vi "Initialization VI.vi"(8 "error in (no error)":errorcluster, 10 "Custom XML":string, 11 "Device Item Ref in":T1 format="%.0x") -> (0 "error out":errorcluster, 3 "Device Item Ref out":T1 format="%.0x")   [LabVIEW 2015, in "DMM-SWITCH-ScanList System Explorer.lvlib"]
uses:
  DMM-SWITCH-ScanList System Explorer.lvlib
  <vilib>/NI Veristand/Custom Device API/Custom Device Item Ref.ctl
  <instrlib>/niDMM/nidmm.llb/niDMM Function.ctl
  <instrlib>/niDMM/nidmm.llb/niDMM Resolution in Digits.ctl
  <instrlib>/niSwitch/niSwitch.LLB/niSwitch Topologies.ctl
  <instrlib>/niSwitch/niSwitch.LLB/niSwitch Trigger Input.ctl
  <instrlib>/niSwitch/niSwitch.LLB/niSwitch Scan Advanced Output.ctl
  <instrlib>/niDMM/nidmm.llb/niDMM Measurement Complete.ctl
  <instrlib>/niDMM/nidmm.llb/niDMM Trigger.ctl
  <vilib>/NI Veristand/Custom Device API/Custom Device Channel.ctl
  <vilib>/NI Veristand/Custom Device API/Custom Device Channel Type.ctl
  Shared/Constants.vi
  <vilib>/NI Veristand/Custom Device API/Custom Device API.lvlib
  Shared/DMM-SWITCH-ScanList Shared.lvlib
  <vilib>/NI/Configuration Framework/serializable configuration/NISE_CEF_serializable configuration.lvclass
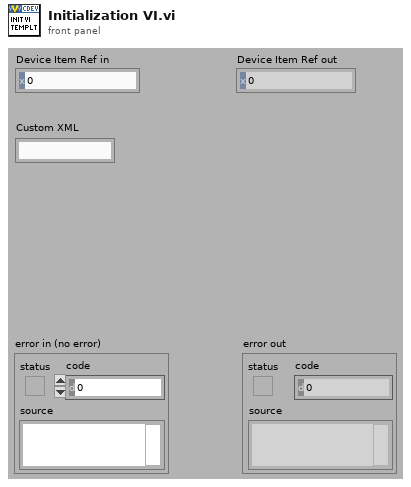
[diagram p1: front panel]
types:
  T1 = typedef "Custom Device API.lvlib/Custom Device Item Ref.ctl" = u64
  T2 = typedef "niDMM Trigger.ctl" = enum16{"Immediate", "External", "TTL 0", "TTL 1", "TTL 2", "TTL 3", "TTL 4", "TTL 5", "TTL 6", "Software", "TTL 7", "PXI Star", "LBR Trig 1", "Aux Trig 1"}
  T3 = typedef "niDMM Measurement Complete.ctl" = enum16{"None", "External", "TTL 0", "TTL 1", "TTL 2", "TTL 3", "TTL 4", "TTL 5", "TTL 6", "TTL 7", "LBR Trig 0"}
  T4 = typedef "niSwitch Scan Advanced Output.ctl" = enum16{"None", "External", "TTL0", "TTL1", "TTL2", "TTL3", "TTL4", "TTL5", "TTL6", "TTL7", "ECL0", "ECL1", "PXI Star", "Rear Connector", "Front Connector", "Rear Connector Module 1", "Rear Connector Module 2", "Rear Connector Module 3", "Rear Connector Module 4", "Rear Connector Module 5", "Rear Connector Module 6", "Rear Connector Module 7", "Rear Connector Module 8", "Rear Connector Module 9", "Rear Connector Module 10", "Rear Connector Module 11", "Rear Connector Module 12", "Front Connector Module 1", "Front Connector Module 2", "Front Connector Module 3", "Front Connector Module 4", "Front Connector Module 5", "Front Connector Module 6", "Front Connector Module 7", "Front Connector Module 8", "Front Connector Module 9", "Front Connector Module 10", "Front Connector Module 11", "Front Connector Module 12"}
  T5 = typedef "niSwitch Trigger Input.ctl" = enum16{"Immediate", "External", "TTL0", "TTL1", "TTL2", "TTL3", "TTL4", "TTL5", "TTL6", "TTL7", "ECL0", "ECL1", "PXI Star", "Software Trigger Function", "Rear Connector", "Front Connector", "Rear Connector of Module 1", "Rear Connector of Module 2", "Rear Connector of Module 3", "Rear Connector of Module 4", "Rear Connector of Module 5", "Rear Connector of Module 6", "Rear Connector of Module 7", "Rear Connector of Module 8", "Rear Connector of Module 9", "Rear Connector of Module 10", "Rear Connector of Module 11", "Rear Connector of Module 12", "Front Connector of Module 1", "Front Connector of Module 2", "Front Connector of Module 3", "Front Connector of Module 4", "Front Connector of Module 5", "Front Connector of Module 6", "Front Connector of Module 7", "Front Connector of Module 8", "Front Connector of Module 9", "Front Connector of Module 10", "Front Connector of Module 11", "Front Connector of Module 12"}
  T6 = typedef "niDMM Function.ctl" = enum16{"DC Volts", "AC Volts", "DC Current", "AC Current", "2-wire Resistance", "4-wire Resistance", "Diode", "Frequency", "Period", "AC Volts DC Coupled", "Capacitance", "Inductance", "Temperature"}
  T7 = typedef "niSwitch Topologies.ctl" = string
  T8 = typedef "niDMM Resolution in Digits.ctl" = dbl
  T9 = typedef "Custom Device API.lvlib/Custom Device Channel.ctl" = cluster{"Type":T10, "Units":string, "Default Value":dbl, "Faultable":bool, "Scalable":bool}
  T10 = typedef "Custom Device API.lvlib/Custom Device Channel Type.ctl" = enum16{"Input", "Output"}
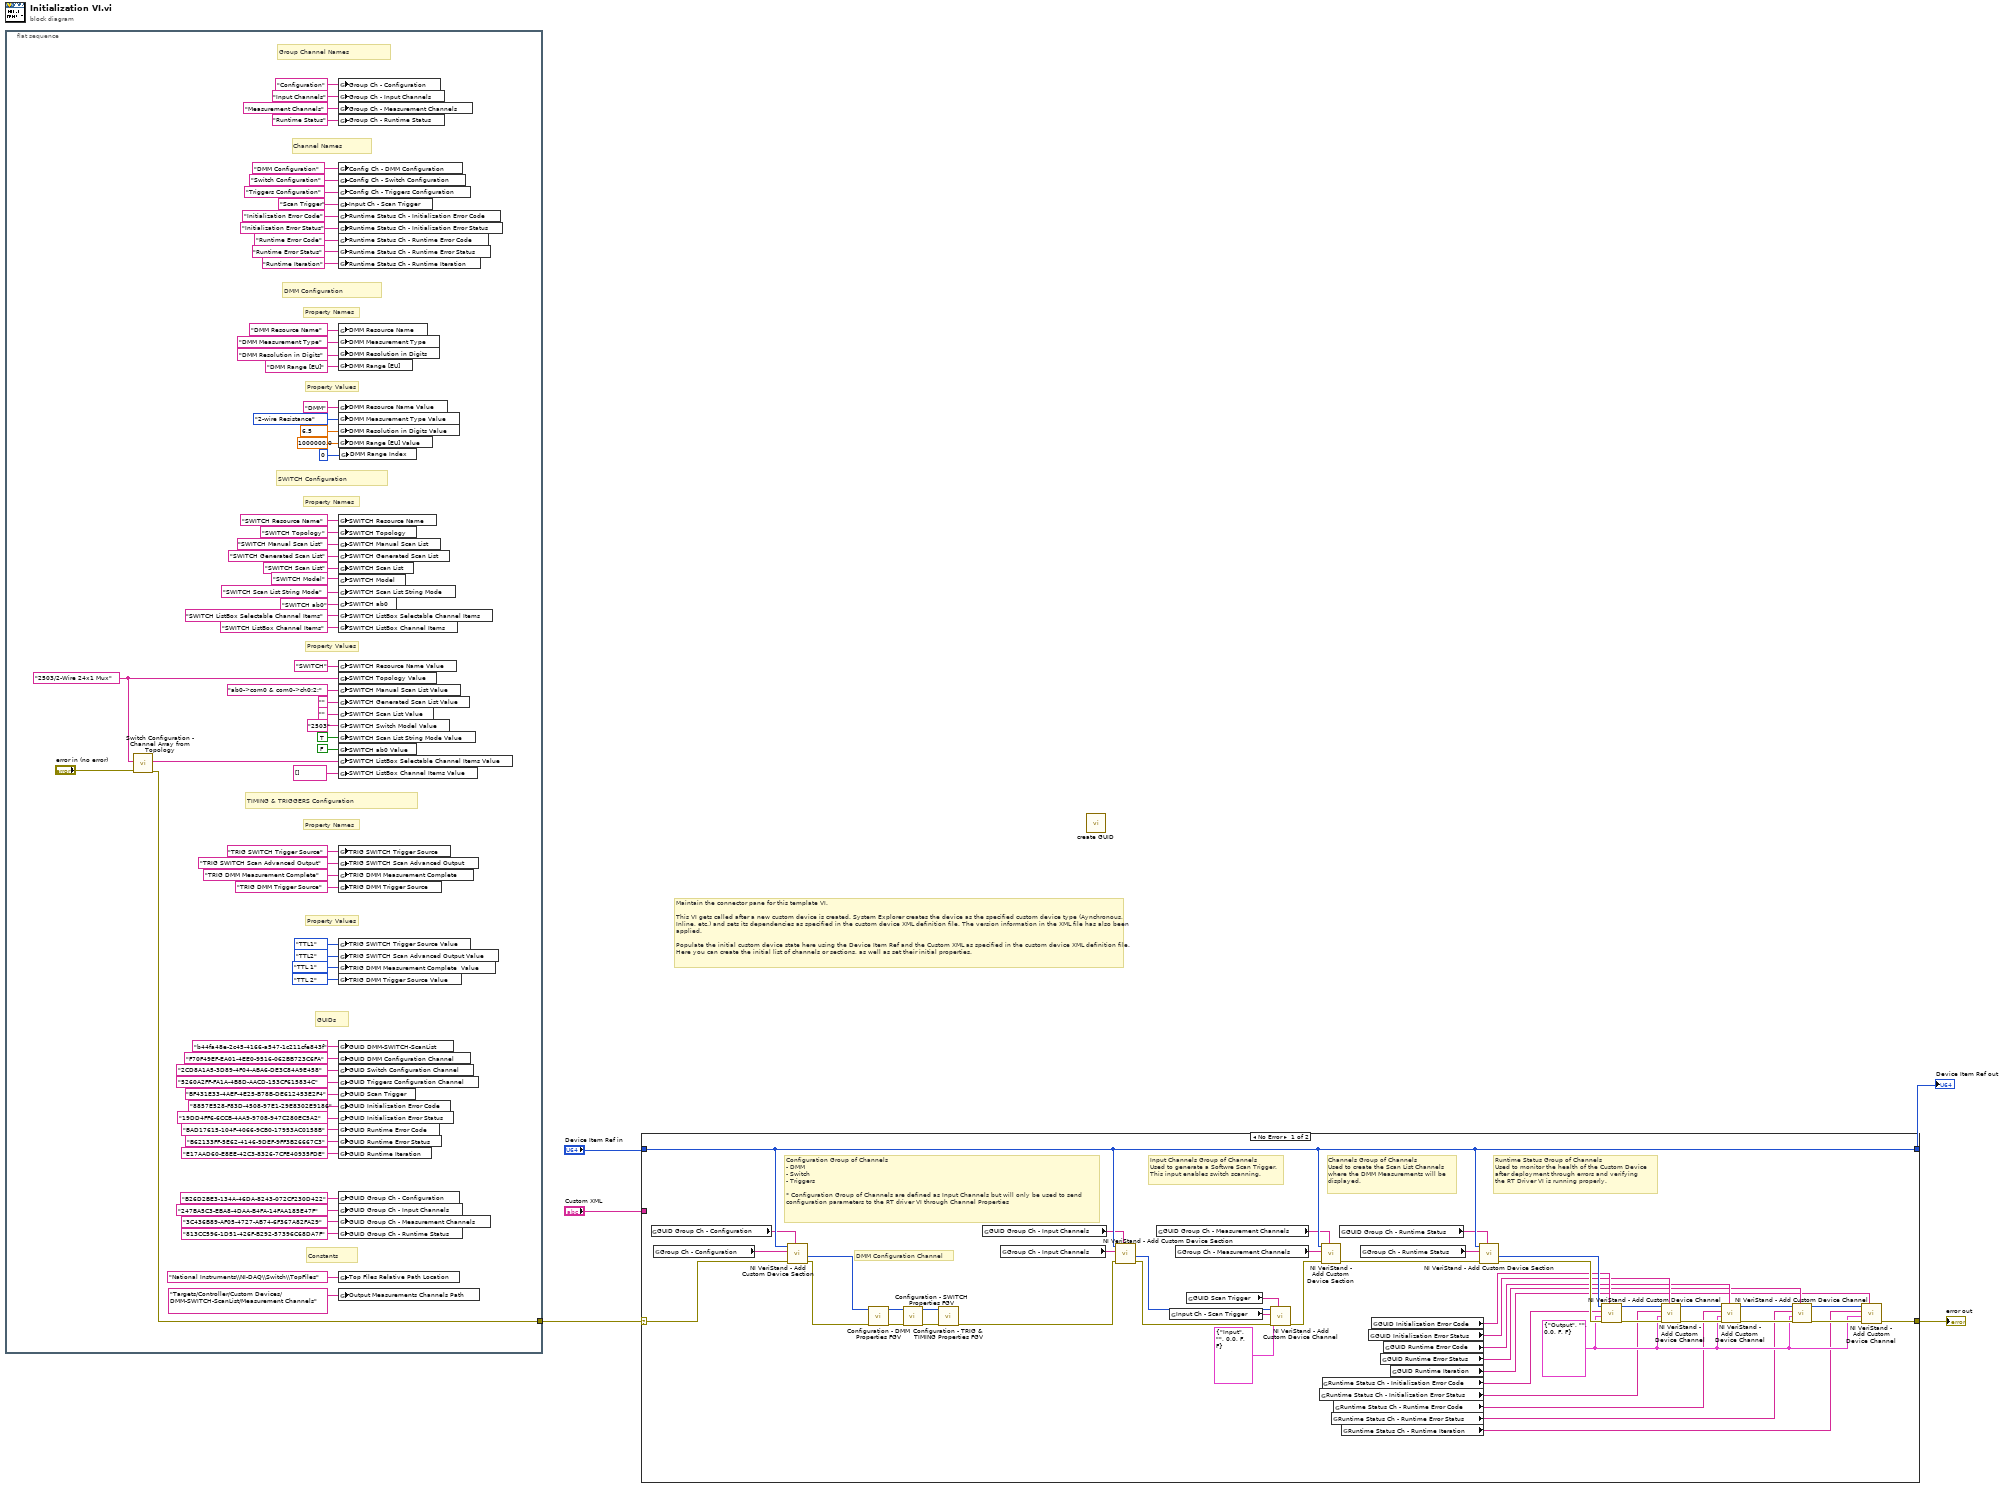
[diagram p0: block diagram]
diagram:
  # "Maintain the connector pane for this template VI.\n\nThis VI gets called after a new custom device is created. System Explorer creates the device as the specified custom device type (Aynchronous, Inline, etc.) and sets its dependencies as specified in the custom device XML definition file. The version information in the XML file has also been applied.\n\nPopulate the initial custom device state here using the Device Item Ref and the Custom XML as specified in the custom device XML definition file. Here you can create the initial list of channels or sections, as well as set their initial properties."
  n1 = flat-sequence {
    tunnel: [w54] -> w5
    frame #0 {
      w55 = T7 "2503/2-Wire 24x1 Mux" ("SWITCH Topology")
      w71 = T8 6.5 items=["3 1/2"=3.5, "4 1/2"=4.5, "5 1/2"=5.5, "6 1/2"=6.5, "7 1/2"=7.5] ("Resolution in Digits")
      # "Channel Names"
      # "Group Channel Names"
      # "Property Values"
      # "Property Names"
      # "Property Values"
      # "Property Names"
      # "Property Values"
      # "Property Names"
      # "Constants"
      # "DMM Configuration"
      # "GUIDs"
      # "TIMING & TRIGGERS Configuration"
      # "SWITCH Configuration"
      n2 = call "Switch Configuration - Channel Array from Topology.vi"("error in (no error)"="error in (no error)", "Selected Mux Topology"=w55) -> ("error out"=w54:errorcluster, "Channel Array Out"=w53:string[])  [unwired: 8 in]
      n3 = global write "Constants.vi" "Group Ch - Configuration"("Configuration" ("Group Ch - Configuration")) -> ()
      n4 = global write "Constants.vi" "Group Ch - Input Channels"("Input Channels" ("Group Ch - Input Channels")) -> ()
      n5 = global write "Constants.vi" "Group Ch - Measurement Channels"("Measurement Channels" ("Group Ch - Measurement Channels")) -> ()
      n6 = global write "Constants.vi" "Group Ch - Runtime Status"("Runtime Status" ("Group Ch - Runtime Status")) -> ()
      n7 = global write "Constants.vi" "Config Ch - DMM Configuration"("DMM Configuration" ("Group Ch - Configuration")) -> ()
      n8 = global write "Constants.vi" "Config Ch - Switch Configuration"("Switch Configuration" ("Group Ch - Input Channels")) -> ()
      n9 = global write "Constants.vi" "Config Ch - Triggers Configuration"("Triggers Configuration" ("Group Ch - Measurement Channels")) -> ()
      n10 = global write "Constants.vi" "Input Ch - Scan Trigger"("Scan Trigger" ("Group Ch - Runtime Status")) -> ()
      n11 = global write "Constants.vi" "Runtime Status Ch - Initialization Error Code"("Initialization Error Code" ("Group Ch - Configuration")) -> ()
      n12 = global write "Constants.vi" "Runtime Status Ch - Initialization Error Status"("Initialization Error Status" ("Group Ch - Input Channels")) -> ()
      n13 = global write "Constants.vi" "Runtime Status Ch - Runtime Error Code"("Runtime Error Code" ("Group Ch - Measurement Channels")) -> ()
      n14 = global write "Constants.vi" "Runtime Status Ch - Runtime Error Status"("Runtime Error Status" ("Group Ch - Runtime Status")) -> ()
      n15 = global write "Constants.vi" "Runtime Status Ch - Runtime Iteration"("Runtime Iteration" ("Group Ch - Runtime Status")) -> ()
      n16 = global write "Constants.vi" "DMM Resource Name"("DMM Resource Name" ("DMM Resource Name")) -> ()
      n17 = global write "Constants.vi" "DMM Measurement Type"("DMM Measurement Type" ("DMM Measurement Type")) -> ()
      n18 = global write "Constants.vi" "DMM Resolution in Digits"("DMM Resolution in Digits" ("DMM Resolution in Digits")) -> ()
      n19 = global write "Constants.vi" "DMM Range [EU]"("DMM Range [EU]" ("DMM Range [EU]")) -> ()
      n20 = global write "Constants.vi" "DMM Resource Name Value"("DMM" ("Value")) -> ()
      n21 = global write "Constants.vi" "DMM Measurement Type Value"(niDMM_Function."2-wire Resistance" ("Function")) -> ()
      n22 = global write "Constants.vi" "DMM Resolution in Digits Value"(w71) -> ()
      n23 = global write "Constants.vi" "DMM Range [EU] Value"(1000000.0 ("DMM Range [EU] Value")) -> ()
      n24 = global write "Constants.vi" "SWITCH Resource Name"("SWITCH Resource Name" ("SWITCH Resource Name")) -> ()
      n25 = global write "Constants.vi" "SWITCH Topology"("SWITCH Topology" ("SWITCH Topology")) -> ()
      n26 = global write "Constants.vi" "SWITCH Manual Scan List"("SWITCH Manual Scan List" ("SWITCH Manual Scan List")) -> ()
      n27 = global write "Constants.vi" "SWITCH Generated Scan List"("SWITCH Generated Scan List" ("SWITCH Generated Scan List")) -> ()
      n28 = global write "Constants.vi" "SWITCH Scan List"("SWITCH Scan List" ("SWITCH Scan List")) -> ()
      n29 = global write "Constants.vi" "SWITCH Model"("SWITCH Model" ("SWITCH Switch Model")) -> ()
      n30 = global write "Constants.vi" "SWITCH Scan List String Mode"("SWITCH Scan List String Mode" ("SWITCH Scan List String Mode")) -> ()
      n31 = global write "Constants.vi" "SWITCH ab0"("SWITCH ab0" ("SWITCH ab0")) -> ()
      n32 = global write "Constants.vi" "SWITCH ListBox Selectable Channel Items"("SWITCH ListBox Selectable Channel Items" ("SWITCH ListBox Selectable Channel Items")) -> ()
      n33 = global write "Constants.vi" "SWITCH ListBox Channel Items"("SWITCH ListBox Channel Items" ("SWITCH ListBox Channel Items")) -> ()
      n34 = global write "Constants.vi" "SWITCH Resource Name Value"("SWITCH" ("SWITCH Resource Name")) -> ()
      n35 = global write "Constants.vi" "SWITCH Topology Value"(w55) -> ()
      n36 = global write "Constants.vi" "SWITCH Manual Scan List Value"("ab0->com0 & com0->ch0:2;" ("SWITCH Manual Scan List")) -> ()
      n37 = global write "Constants.vi" "SWITCH Generated Scan List Value"("" ("SWITCH Generated Scan List")) -> ()
      n38 = global write "Constants.vi" "SWITCH Scan List Value"("" ("SWITCH Scan List")) -> ()
      n39 = global write "Constants.vi" "SWITCH Switch Model Value"("2503" ("SWITCH Switch Model")) -> ()
      n40 = global write "Constants.vi" "SWITCH Scan List String Mode Value"(TRUE ("SWITCH Scan List String Mode")) -> ()
      n41 = global write "Constants.vi" "SWITCH ab0 Value"(FALSE ("SWITCH ab0")) -> ()
      n42 = global write "Constants.vi" "SWITCH ListBox Selectable Channel Items Value"(w53) -> ()
      n43 = global write "Constants.vi" "SWITCH ListBox Channel Items Value"(string[] [] ("SWITCH ListBox Channel Items")) -> ()
      n44 = global write "Constants.vi" "TRIG SWITCH Trigger Source"("TRIG SWITCH Trigger Source" ("TRIG SWITCH Trigger Source")) -> ()
      n45 = global write "Constants.vi" "TRIG SWITCH Scan Advanced Output"("TRIG SWITCH Scan Advanced Output" ("TRIG SWITCH Scan Advanced Output")) -> ()
      n46 = global write "Constants.vi" "TRIG DMM Measurement Complete"("TRIG DMM Measurement Complete" ("TRIG DMM Measurement Complete")) -> ()
      n47 = global write "Constants.vi" "TRIG DMM Trigger Source"("TRIG DMM Trigger Source" ("TRIG DMM Trigger Source")) -> ()
      n48 = global write "Constants.vi" "TRIG SWITCH Trigger Source Value"(niSwitch_Trigger_Input."TTL1" ("TRIG SWITCH Trigger Source")) -> ()
      n49 = global write "Constants.vi" "TRIG SWITCH Scan Advanced Output Value"(niSwitch_Scan_Advanced_Output."TTL2" ("TRIG SWITCH Scan \nAdvanced Output")) -> ()
      n50 = global write "Constants.vi" "TRIG DMM Measurement Complete  Value"(niDMM_Measurement_Complete."TTL 1" ("TRIG DMM Measurement \nComplete Destination")) -> ()
      n51 = global write "Constants.vi" "TRIG DMM Trigger Source Value"(niDMM_Trigger."TTL 2" ("TRIG DMM Trigger Source")) -> ()
      n52 = global write "Constants.vi" "GUID DMM-SWITCH-ScanList"("b44fa48e-2c45-4166-a547-1c211cfe843f" ("GUID DMM-SWITCH-ScanList")) -> ()
      n53 = global write "Constants.vi" "GUID DMM Configuration Channel"("F70F49EF-EA01-4EE0-9516-062BB723C6FA" ("GUID DMM Configuration Channel")) -> ()
      n54 = global write "Constants.vi" "GUID Switch Configuration Channel"("2CD8A1A5-3D89-4F04-ABA6-DE3C84A9E458" ("GUID Switch Configuration Channel")) -> ()
      n55 = global write "Constants.vi" "GUID Triggers Configuration Channel"("5260A2FF-FA1A-4B8D-AACD-153CF615834C" ("GUID Triggers Configuration Channel")) -> ()
      n56 = global write "Constants.vi" "GUID Scan Trigger"("BF431E33-4AEF-4E25-B78B-DE612453E2F4" ("GUID DMM-SWITCH-ScanList")) -> ()
      n57 = global write "Constants.vi" "GUID Initialization Error Code"("8857E528-F83D-4508-97E1-29E8302E9186" ("GUID DMM Configuration Channel")) -> ()
      n58 = global write "Constants.vi" "GUID Initialization Error Status"("19DD4FF6-6CCB-4AA9-9708-947C280EC5A2" ("GUID Switch Configuration Channel")) -> ()
      n59 = global write "Constants.vi" "GUID Runtime Error Code"("BAD17615-104F-4066-9CB0-17953AC0158B" ("GUID Triggers Configuration Channel")) -> ()
      n60 = global write "Constants.vi" "GUID Runtime Error Status"("B62133FF-5E62-4146-9DEF-9FF3B26667C3" ("GUID Triggers Configuration Channel")) -> ()
      n61 = global write "Constants.vi" "GUID Runtime Iteration"("E17AAD60-E8EE-42C3-8326-7CFE40935FDE" ("GUID Triggers Configuration Channel")) -> ()
      n62 = global write "Constants.vi" "GUID Group Ch - Configuration"("B26D2BE3-134A-46DA-8243-072CF230D422" ("GUID Triggers Configuration Channel")) -> ()
      n63 = global write "Constants.vi" "GUID Group Ch - Input Channels"("247BA5C3-EBA8-4DAA-B4FA-14FAA185E47F" ("GUID Triggers Configuration Channel")) -> ()
      n64 = global write "Constants.vi" "GUID Group Ch - Measurement Channels"("3C436B89-AF05-4727-AB74-6F367A82FA29" ("GUID Triggers Configuration Channel")) -> ()
      n65 = global write "Constants.vi" "GUID Group Ch - Runtime Status"("813CC596-1D51-426F-B292-57396C68DA7F" ("GUID Triggers Configuration Channel")) -> ()
      n66 = global write "Constants.vi" "Top Files Relative Path Location"("National Instruments\\NI-DAQ\\Switch\\TopFiles" ("Top Files Relative Path Location")) -> ()
      n67 = global write "Constants.vi" "Output Measurements Channels Path"("Targets/Controller/Custom Devices/DMM-SWITCH-ScanList/Measurement Channels" ("Output Measurements Channels Path")) -> ()
      n68 = global write "Constants.vi" "DMM Range Index"(u16 0 ("DMM Range Index")) -> ()
    }
  }
  n69 = case shown="No Error" w5 {
    selector: w5 -> [w115 w121]
    tunnel: [w91 w121] -> w1
    tunnel: [w96 w120] -> w3
    tunnel: "Device Item Ref in" -> [w96 w120]
    tunnel: "Custom XML" -> [_ _]
    frame No Error {
      w102 = T9 {"Type"=enum."Output", "Units"="", "Default Value"=0.0, "Faultable"=FALSE, "Scalable"=FALSE} ("Channel")
      # "Input Channels Group of Channels\nUsed to generate a Softwre Scan Trigger.\nThis input enables switch scanning."
      # "Runtime Status Group of Channels\nUsed to monitor the health of the Custom Device\nafter deployment through errors and verifying \nthe RT Driver VI is running properly."
      # "Channels Group of Channels\nUsed to create the Scan List Channels\nwhere the DMM Measurements will be\ndisplayed."
      # "DMM Configuration Channel"
      # "Configuration Group of Channels\n- DMM\n- Switch\n- Triggers\n\n* Configuration Group of Channels are defined as Input Channels but will only be used to send \nconfiguration parameters to the RT driver VI through Channel Properties"
      n70 = global read "Constants.vi" "GUID Group Ch - Configuration"() -> (w83:string)
      n71 = global read "Constants.vi" "Group Ch - Configuration"() -> (w84:string)
      n72 = call <vilib>:"NI VeriStand - Add Custom Device Section.vi"("GUID (Default Section)"=w83, "error in (no error)"=w115, "Section Name"=w84, "Parent Ref in"=w96) -> ("error out"=w119:errorcluster, "Section Ptr"=w118:T1)  [unwired: 4 in, 2 out]
      n73 = call "Configuration - DMM Properties FGV.vi"("error in (no error)"=w119, "Configuration Group of Channels Ref In"=w118) -> ("error out"=w114:errorcluster, "Configuration Group of Channels Ref Out"=w117:T1)  [unwired: 8 in]
      n74 = call "Configuration - SWITCH Properties FGV.vi"("error in (no error)"=w114, "Parent Ref in"=w117) -> ("error out"=w113:errorcluster, "Parent Ref out"=w116:T1)  [unwired: 8 in]
      n75 = call "Configuration - TRIG & TIMING Properties FGV.vi"("error in (no error)"=w113, "Parent Ref in"=w116) -> ("error out"=w98:errorcluster)  [unwired: 9 in]
      n76 = global read "Constants.vi" "GUID Group Ch - Input Channels"() -> (w82:string)
      n77 = global read "Constants.vi" "Group Ch - Input Channels"() -> (w94:string)
      n78 = call <vilib>:"NI VeriStand - Add Custom Device Section.vi"("GUID (Default Section)"=w82, "error in (no error)"=w98, "Section Name"=w94, "Parent Ref in"=w96) -> ("error out"=w100:errorcluster, "Section Ptr"=w101:T1)  [unwired: 4 in, 2 out]
      n79 = global read "Constants.vi" "GUID Group Ch - Measurement Channels"() -> (w81:string)
      n80 = global read "Constants.vi" "Input Ch - Scan Trigger"() -> (w90:string)
      n81 = global read "Constants.vi" "Group Ch - Measurement Channels"() -> (w93:string)
      n82 = global read "Constants.vi" "GUID Scan Trigger"() -> (w74:string)
      n83 = call <vilib>:"NI VeriStand - Add Custom Device Channel.vi"("GUID (Default Channel)"=w74, "error in (no error)"=w100, "Channel"=T9 {"Type"=enum."Input", "Units"="", "Default Value"=0.0, "Faultable"=FALSE, "Scalable"=FALSE}, "Channel Name"=w90, "Parent Ref in"=w101) -> ("error out"=w99:errorcluster)  [unwired: 3 in, 3 out]
      n84 = global read "Constants.vi" "Runtime Status Ch - Initialization Error Status"() -> (w88:string)
      n85 = call <vilib>:"NI VeriStand - Add Custom Device Section.vi"("GUID (Default Section)"=w81, "error in (no error)"=w99, "Section Name"=w93, "Parent Ref in"=w96) -> ("error out"=w112:errorcluster)  [unwired: 4 in, 3 out]
      n86 = global read "Constants.vi" "Runtime Status Ch - Initialization Error Code"() -> (w89:string)
      n87 = global read "Constants.vi" "Runtime Status Ch - Runtime Error Status"() -> (w86:string)
      n88 = global read "Constants.vi" "Runtime Status Ch - Runtime Error Code"() -> (w87:string)
      n89 = global read "Constants.vi" "GUID Group Ch - Runtime Status"() -> (w80:string)
      n90 = global read "Constants.vi" "Runtime Status Ch - Runtime Iteration"() -> (w85:string)
      n91 = global read "Constants.vi" "Group Ch - Runtime Status"() -> (w92:string)
      n92 = global read "Constants.vi" "GUID Initialization Error Status"() -> (w78:string)
      n93 = global read "Constants.vi" "GUID Initialization Error Code"() -> (w79:string)
      n94 = global read "Constants.vi" "GUID Runtime Error Status"() -> (w76:string)
      n95 = global read "Constants.vi" "GUID Runtime Error Code"() -> (w77:string)
      n96 = global read "Constants.vi" "GUID Runtime Iteration"() -> (w75:string)
      n97 = call <vilib>:"NI VeriStand - Add Custom Device Section.vi"("GUID (Default Section)"=w80, "error in (no error)"=w112, "Section Name"=w92, "Parent Ref in"=w96) -> ("error out"=w104:errorcluster, "Section Ptr"=w103:T1)  [unwired: 4 in, 2 out]
      n98 = call <vilib>:"NI VeriStand - Add Custom Device Channel.vi"("GUID (Default Channel)"=w79, "error in (no error)"=w104, "Channel"=w102, "Channel Name"=w89, "Parent Ref in"=w103) -> ("error out"=w111:errorcluster, "Parent Ref out"=w95:T1)  [unwired: 3 in, 2 out]
      n99 = call <vilib>:"NI VeriStand - Add Custom Device Channel.vi"("GUID (Default Channel)"=w78, "error in (no error)"=w111, "Channel"=w102, "Channel Name"=w88, "Parent Ref in"=w95) -> ("error out"=w109:errorcluster, "Parent Ref out"=w110:T1)  [unwired: 3 in, 2 out]
      n100 = call <vilib>:"NI VeriStand - Add Custom Device Channel.vi"("GUID (Default Channel)"=w77, "error in (no error)"=w109, "Channel"=w102, "Channel Name"=w87, "Parent Ref in"=w110) -> ("error out"=w107:errorcluster, "Parent Ref out"=w108:T1)  [unwired: 3 in, 2 out]
      n101 = call <vilib>:"NI VeriStand - Add Custom Device Channel.vi"("GUID (Default Channel)"=w76, "error in (no error)"=w107, "Channel"=w102, "Channel Name"=w86, "Parent Ref in"=w108) -> ("error out"=w106:errorcluster, "Parent Ref out"=w105:T1)  [unwired: 3 in, 2 out]
      n102 = call <vilib>:"NI VeriStand - Add Custom Device Channel.vi"("GUID (Default Channel)"=w75, "error in (no error)"=w106, "Channel"=w102, "Channel Name"=w85, "Parent Ref in"=w105) -> ("error out"=w91:errorcluster)  [unwired: 3 in, 3 out]
    }
    frame Error {
    }
  }
  "error out" <- w1
  "Device Item Ref out" <- w3
  n103 = call <vilib>:"create GUID.vi"() -> ()  [unwired: 10 in, 2 out]
